vi "Array(2D)_to_File.vi"(5 "path (use dialog)":path=path "C:/misc/LabVIEW/FILES/*.psv", 9 "Array":dbl[][](array[numeric]) format="%_8f") -> (6 "Saved String":string)   [LabVIEW 2014]
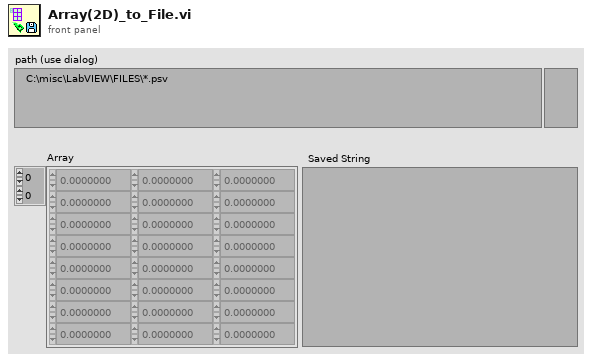
[diagram p1: front panel]
types:
  T1 = enum16{"open", "replace", "create", "open or create", "replace or create", "replace or create with confirmation"}
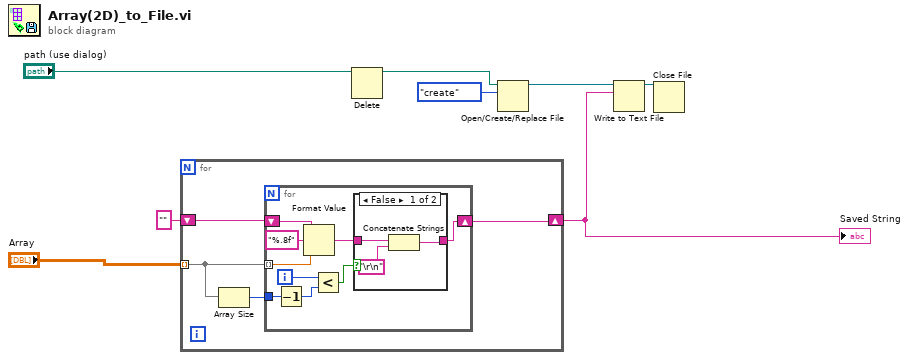
[diagram p0: block diagram]
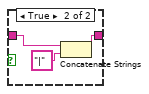
[diagram p2: hidden frame]
diagram:
  n1 = for {
    tunnel: "Array" -> [w11] mode=indexing
    shift-right: [w9] -> w8
    shift-left: "" -> [w12]
    n2 = Array Size(array=w11) -> (size(s)=w10:i32)
    n3 = for {
      tunnel: w11 -> [w21] mode=indexing
      shift-right: [w13] -> w9
      shift-left: w12 -> [w20]
      tunnel: w10 -> [w16]
      i -> [w15]
      n4 = Decrement(x=w16) -> (x-1=w17:i32)
      n5 = Format Value(string ("")=w20, format string="%.8f", value (0)=w21) -> (output string=w14:string)
      n6 = Less?(x=w15, y=w17) -> (x < y?=w18:bool)
      n7 = case shown="False" w18 {
        tunnel: [w24 w26] -> w13
        tunnel: w14 -> [w23 w25]
        frame False {
          n8 = Concatenate Strings(w23, "\r\n") -> (w24:string)
        }
        frame True {
          n9 = Concatenate Strings(w25, "|") -> (w26:string)
        }
      }
    }
  }
  "Saved String" <- w8
  n10 = Delete(path (use dialog)="path (use dialog)") -> (deleted path=w7:path)  [unwired: 4 in, 2 out]
  n11 = Open/Create/Replace File(file path (use dialog)=w7, operation (0:open)=T1."create") -> (refnum out=w4:refnum<file>)  [unwired: 1 in, 5 out]
  n12 = Write to Text File(file (use dialog)=w4, text=w8) -> (refnum out=w5:refnum<file>)  [unwired: 2 in, 2 out]
  n13 = Close File(refnum=w5) -> ()  [unwired: 1 in, 2 out]
